vi "Read Flat Configuration.vi"(8 "error in (no error)":errorcluster, 11 "CIFTemplateNode in":refnum<class "CIFCorePlugin.lvclass">) -> (0 "error out":errorcluster, 2 "Configuration":variant, 3 "CIFTemplateNode out":refnum<class "CIFCorePlugin.lvclass">)   [LabVIEW 2021, in "CIFCorePlugin.lvclass"]
uses:
  CIFCorePlugin.lvclass
  CIFCorePlugin.lvclass/CIFCorePlugin.ctl
  CIFCoreOOB/OOB_Rx/CIFCoreOOB_Rx.lvclass
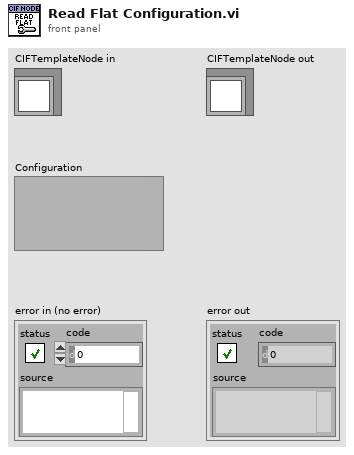
[diagram p1: front panel]
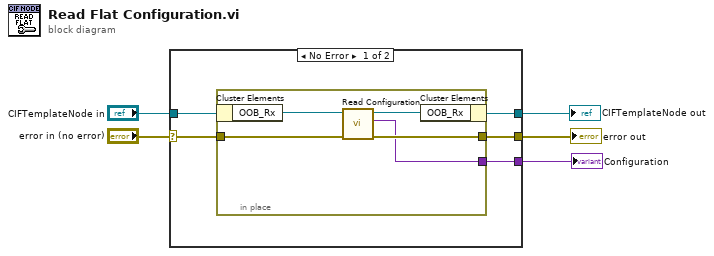
[diagram p0: block diagram]
diagram:
  n1 = case shown="No Error" "error in (no error)" {
    selector: "error in (no error)" -> [w9 w16]
    tunnel: [w8 w16] -> w4
    tunnel: [w7 w17] -> w2
    tunnel: "CIFTemplateNode in" -> [w10 w17]
    tunnel: [w6 _] -> w1
    frame No Error {
      n2 = in-place {
        in-place-border: w9 -> [w13]
        in-place-border: [w12] -> w8
        in-place-border: [w11] -> w6
        n3 = in-place-cluster #1(w10) -> ("OOB_Rx"=w15:refnum<class "CIFCoreOOB_Rx.lvclass">)
        n4 = call "Read Configuration.vi"("error in"=w13, "CoreOOB_Rx in"=w15) -> ("error out"=w12:errorcluster, "Configuration Data"=w11:variant, "CoreOOB_Rx out"=w14:refnum<class "CIFCoreOOB_Rx.lvclass">)  [unwired: 7 in]
        n5 = in-place-cluster #1("OOB_Rx"=w14) -> (w7:refnum<class "CIFCorePlugin.lvclass">)
      }
    }
    frame Error {
    }
  }
  "error out" <- w4
  "CIFTemplateNode out" <- w2
  "Configuration" <- w1
